vi "Set ESP Variable.vi"   [LabVIEW 2017, in "NI_WebServices.lvlib"]
doc: "LabVIEW no longer supports this VI. Replace this VI with the Set ESP Variable VI of the same name from the Output palette.\n\nSets variables to be visible in an ESP scripting template. You can access these variables from the form variables in the ESP template. Refer to the Scripting in LabVIEW Web Services topic at ni.com/zone for more information about using scripting with Web services. The data type you wire to the <B>value</B> input determines the polymorphic instance to use."
uses:
  <vilib>/wsapi/NI_WebServices.lvlib
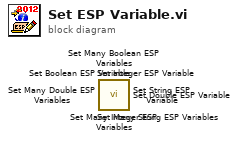
[diagram p0: block diagram]
diagram:
  n1 = call <vilib>:"Set Many Integer ESP Variables.vi"() -> ()  [unwired: 10 in, 2 out]
  n2 = call <vilib>:"Set Integer ESP Variable.vi"() -> ()  [unwired: 10 in, 2 out]
  n3 = call <vilib>:"Set Many Double ESP Variables.vi"() -> ()  [unwired: 10 in, 2 out]
  n4 = call <vilib>:"Set Double ESP Variable.vi"() -> ()  [unwired: 10 in, 2 out]
  n5 = call <vilib>:"Set Many Boolean ESP Variables.vi"() -> ()  [unwired: 10 in, 2 out]
  n6 = call <vilib>:"Set Boolean ESP Variable.vi"() -> ()  [unwired: 10 in, 2 out]
  n7 = call <vilib>:"Set Many String ESP Variables.vi"() -> ()  [unwired: 10 in, 2 out]
  n8 = call <vilib>:"Set String ESP Variable.vi"() -> ()  [unwired: 10 in, 2 out]
